vi "Something.vi"(8 "error in (no error)":errorcluster, 11 "Multiplexer_Opmux in":refnum<class "Multiplexer_Opmux.lvclass">) -> (0 "error out":errorcluster, 3 "Multiplexer_Opmux out":refnum<class "Multiplexer_Opmux.lvclass">)   [LabVIEW 2014, in "Multiplexer_Opmux.lvclass"]
uses:
  Multiplexer_Opmux.lvclass
  Multiplexer_Opmux.lvclass/Multiplexer_Opmux.ctl
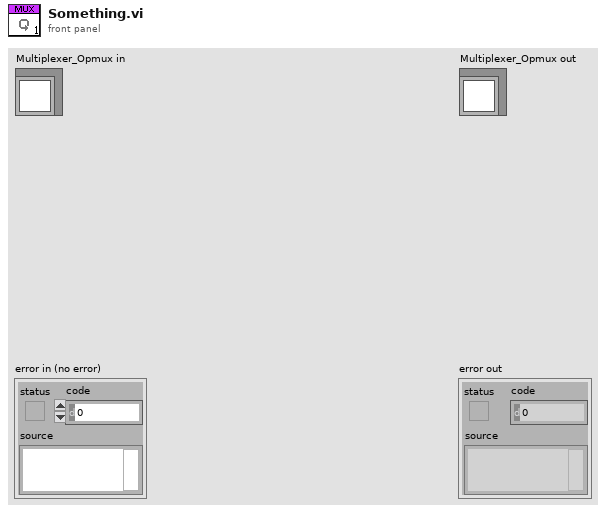
[diagram p1: front panel]
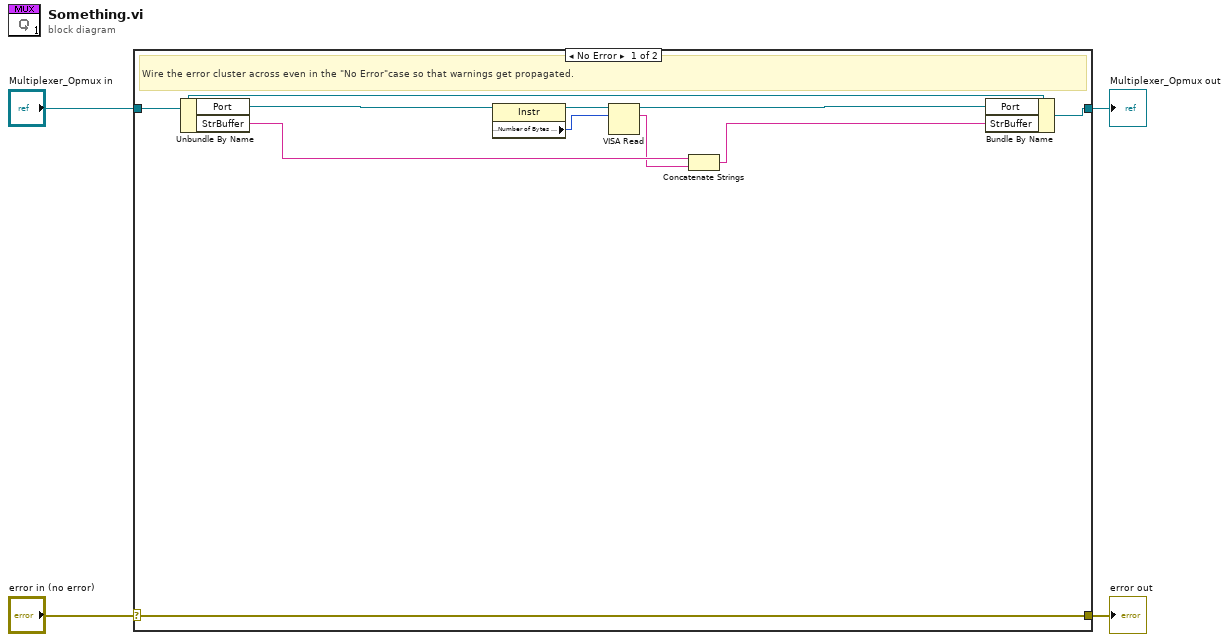
[diagram p0: block diagram]
diagram:
  n1 = case shown="No Error" "error in (no error)" {
    selector: "error in (no error)" -> [w14 w16]
    tunnel: [w14 w16] -> w3
    tunnel: [w13 w15] -> w1
    tunnel: "Multiplexer_Opmux in" -> [w12 w15]
    frame No Error {
      # "Wire the error cluster across even in the \"No Error\"case so that warnings get propagated."
      n2 = Unbundle By Name(w12) -> ("Port"=w9:refnum<visa-resource-name>, "StrBuffer"=w7:string)
      n3 = property class="Instr"(reference=w9) -> (reference out=w10:refnum<visa-resource-name>, "Serial Settings:Number of Bytes at Serial Port"=w11:u32)  [unwired: 1 in, 1 out]
      n4 = VISA Read(VISA resource name=w10, byte count=w11) -> (VISA resource name out=w8:refnum<visa-resource-name>, read buffer=w6:string)  [unwired: 1 in, 2 out]
      n5 = Concatenate Strings(w7, w6) -> (w5:string)
      n6 = Bundle By Name(cluster=w12, "Port"=w8, "StrBuffer"=w5) -> (w13:refnum<class "Multiplexer_Opmux.lvclass">)
    }
    frame Error {
    }
  }
  "error out" <- w3
  "Multiplexer_Opmux out" <- w1
